vi "Write Dependencies.vi"(8 "error in (no error)":errorcluster, 10 "Control Experiment":refnum<class "SMO.Control Experiment.lvclass">, 11 "Transport in":refnum<class "SMO.Transport.lvclass">) -> (0 "error out":errorcluster, 3 "Transport out":refnum<class "SMO.Transport.lvclass">)   [LabVIEW 2019, in "SMO.Transport.lvclass"]
uses:
  SMO.Transport.lvclass
  SMO.Control Experiment/SMO.Control Experiment.lvclass
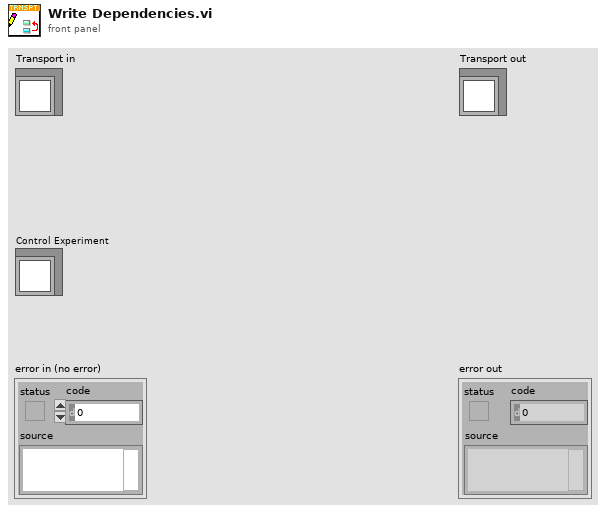
[diagram p1: front panel]
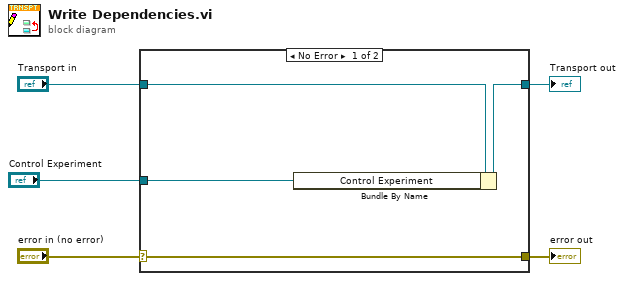
[diagram p0: block diagram]
diagram:
  n1 = case shown="No Error" "error in (no error)" {
    selector: "error in (no error)" -> [w6 w10]
    tunnel: [w6 w10] -> w4
    tunnel: [w8 w11] -> w2
    tunnel: "Transport in" -> [w9 w11]
    tunnel: "Control Experiment" -> [w7 _]
    frame No Error {
      n2 = Bundle By Name(cluster=w9, "Control Experiment"=w7) -> (w8:refnum<class "SMO.Transport.lvclass">)
    }
    frame Error {
    }
  }
  "error out" <- w4
  "Transport out" <- w2
